vi "Drive Controller.vi"(8 "error in":errorcluster) -> ()   [LabVIEW 2019]
doc: "This VI executes continuously carrying out the current operation and responding to updates or new operation requests. It will often contain the timing or control code that is difficult to place directly in TeleOp. This VI generally opens all sensors and motors and isolates the rest of the robot code from knowing implementation details of how the operations are carried out."
uses:
  <vilib>/Rock Robotics/WPI/Framework/Completion Status.ctl
  Drive Setpoints.ctl
  Drive Operations.ctl
  Dawgma Programming Library/Controls/PurePursuit/RobotNeededPathData.ctl
  <vilib>/Rock Robotics/WPI/ThirdParty/REV Robotics/SPARK MAX/Typedef/Spark MAX Sensor Type.ctl
  <vilib>/Rock Robotics/WPI/ThirdParty/REV Robotics/SPARK MAX/Typedef/Spark MAX Idle Mode.ctl
  <vilib>/Rock Robotics/WPI/DriverStation/WPI_DriverStationRobotMode2.ctl
  <vilib>/Rock Robotics/WPI/ThirdParty/REV Robotics/SPARK MAX/Typedef/Spark MAX Control Type.ctl
  Dawgma Programming Library/Controls/PurePursuit/PathFileData.ctl
  Framework/Robot Global Data.vi
  <vilib>/Rock Robotics/Network Tables/NT Write Numeric Array.vi
  <vilib>/Rock Robotics/Network Tables/NT Read Number.vi
  Configuration/Constants.vi
  <vilib>/Rock Robotics/WPI/ThirdParty/Sensors/navX/_Processing Loop/FRIC_navX_Internal_SPI_ProcessingLoop.vi
  <extravilib>/ChannelInstances/Lossy Stream-c(dbl,dbl,dbl,dbl,dbl,c(dbl,dbl)).lvlib
panel:
  in  "R L & A":bool
  out "Graph":cluster{cluster{"x":dbl, "y":dbl}[]}[](graph)
  in  "PurePursuit Gains":T1={"FFV"=0.0055, "FFA"=0.0025, "Vel PID"={"P"=0.0001, "I"=0.0, "D"=0.0}}
  in  "SensorData":T2={"LeftDistance"=3962.033502451172, "RightDistance"=3821.920006201172, "LeftVelocity"=0.0, "RightVelocity"=0.0, "Angle"=-59.4, "Location"={597.0445781606653, 278.6835922961287}}
  in  "Reset PID":bool
  out "Right Motor Out":dbl=0.05499435407574694
  out "Left Motor Out":dbl=0.05499435407574694
  in  "SparkMAX PID":T3={"P"=0.038, "I"=0.0, "D"=0.0, "F"=0.001, "I Zone"=0.0, "Min Output"=-0.8, "Max Output"=0.8}
  in  "Reset Encoders":bool
  in  "Coast?":bool
  in  "Interactive Values":T4={"Operation"=enum."Drive for Distance", "Left Setpoint"=0.2, "Right Setpoint"=-0.2, "Duration"=0.1, "Distance"=200.0, "RobotNeededPathData"={"Path"=[], "MaxVel"=0.0, "MaxAccel"=0.0, "Backwards?"=FALSE, "PointSpacing"=0.0, "LookaheadDist"=0.0, "Speed/Curve"=1.8, "SlowDistanceAtEnd"=12.0, "SlowSpeed"=15.0, "MaxDeAccel"=0.0}, "PathPath"=""} {"RobotNeededPathData"."SlowSpeed" format="%#_13g"; "RobotNeededPathData"."SlowDistanceAtEnd" format="%#_13g"; "RobotNeededPathData"."Speed/Curve" format="%#_13g"}
  in  "Buttons":cluster{"Execute Cmd":bool, "Abort Cmd":bool}
  out "Command Timing":cluster{"Start Time (ms)":u32, "Iterations":i32}={"Start Time (ms)"=608665, "Iterations"=0}
  out "Status":T7
  out "Current\nCmd":string="Started at  13:49:29.041\nDefault: Reserve,  L 0.0, R 0.0, D 0.000000"
  # "Interactive Command: You may fill in the settings for a command\nand schedule it with the Execute button. You can observe and abort\nany command while fine tuning the code for the controller."
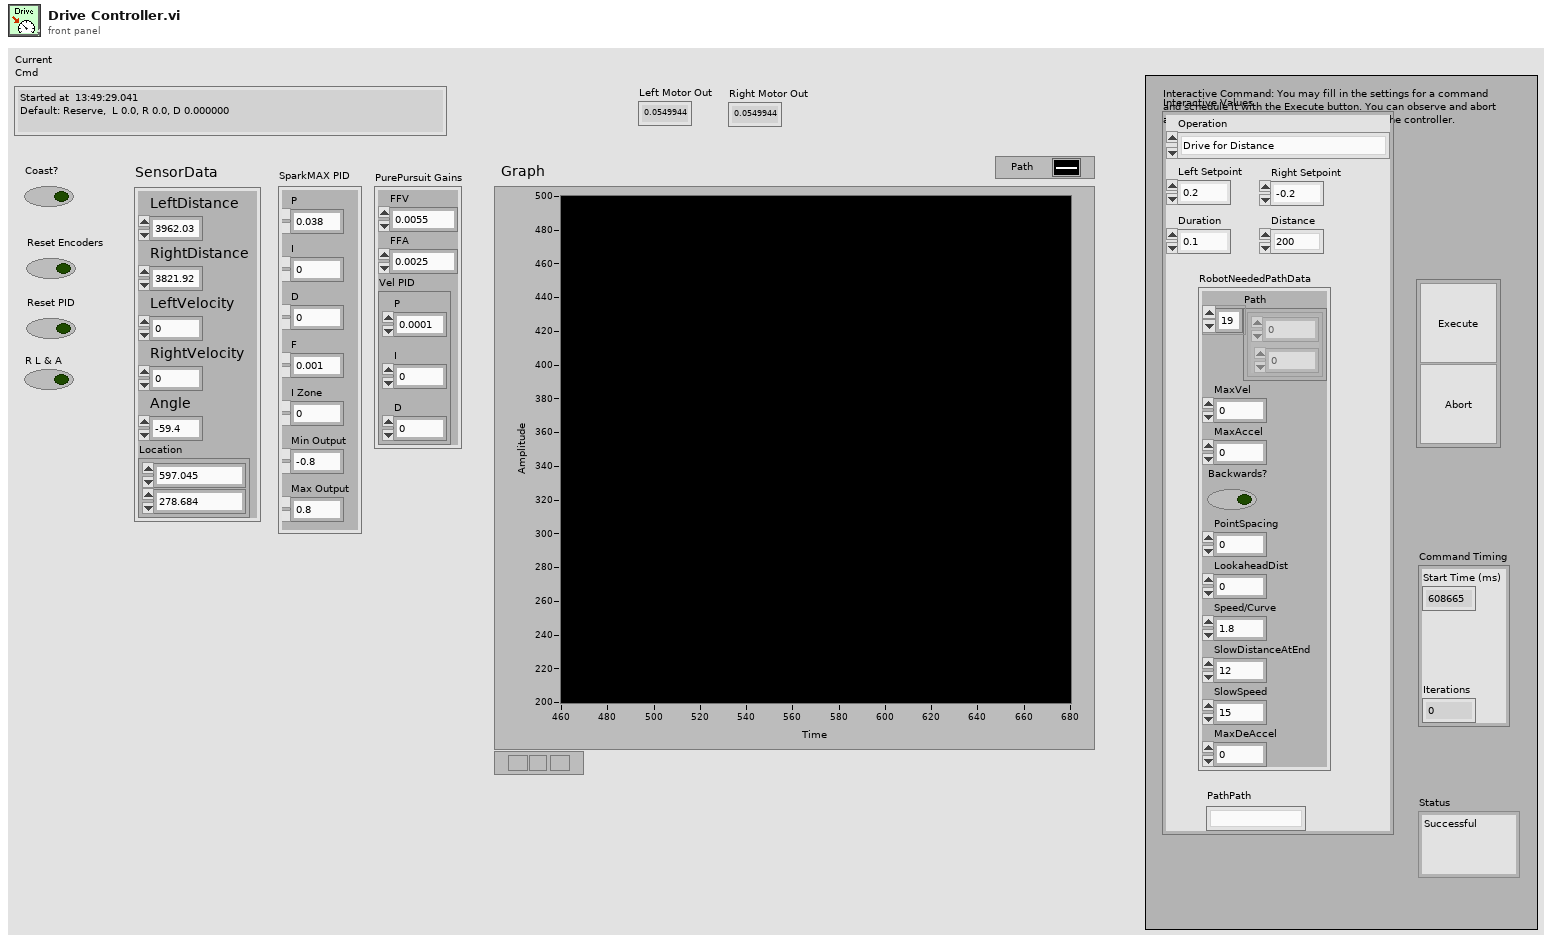
[diagram p1: front panel]
types:
  T1 = cluster{"FFV":dbl, "FFA":dbl, "Vel PID":cluster{"P":dbl, "I":dbl, "D":dbl}}
  T2 = cluster{"LeftDistance":dbl, "RightDistance":dbl, "LeftVelocity":dbl, "RightVelocity":dbl, "Angle":dbl, "Location":cluster{dbl, dbl}}
  T3 = cluster{"P":dbl, "I":dbl, "D":dbl, "F":dbl, "I Zone":dbl, "Min Output":dbl, "Max Output":dbl}
  T4 = typedef "Drive Setpoints.ctl" = cluster{"Operation":T5, "Left Setpoint":dbl, "Right Setpoint":dbl, "Duration":dbl, "Distance":dbl, "RobotNeededPathData":T6, "PathPath":string}
  T5 = typedef "Drive Operations.ctl" = enum16{"Reserve", "Read Current", "Immediate", "Drive for Time", "Drive for Distance", "Drive Path", "Pure Pursuit Test", "Auto Align"}
  T6 = typedef "RobotNeededPathData.ctl" = cluster{"Path":cluster{dbl, dbl}[], "MaxVel":dbl, "MaxAccel":dbl, "Backwards?":bool, "PointSpacing":dbl, "LookaheadDist":dbl, "Speed/Curve":dbl, "SlowDistanceAtEnd":dbl, "SlowSpeed":dbl, "MaxDeAccel":dbl}
  T7 = typedef "Completion Status.ctl" = enum16{"Successful", "Aborted", "Incomplete"}
  T8 = typedef "Spark MAX Idle Mode.ctl" = enum16{"Coast", "Brake"}
  T9 = typedef "Spark MAX Sensor Type.ctl" = enum16{"No Sensor", "Hall Sensor", "Encoder", "-Not Available-", "Analog", "Alternate Encoder"}
  T10 = typedef "WPI_MotorControlDeviceRef.ctl" = cluster{"DeviceStatus":errorcluster, "Type":T11, "PWM":cluster{"PWM Channel":T12, "DeadBand":T13}, "CAN":cluster{"Device Number":u8, "SetOutput VI Ref":variant, "GetOutput VI Ref":variant, "Enable VI Ref":variant, "Disable VI Ref":variant, "Data":variant}, "Invert":bool, "DIO PWM":cluster{"PWM \"Enable\" Channel":T12, "DIOChannel":T14, "PWM Rate":dbl}}
  T11 = typedef "WPI_MotorControlType.ctl" = enum16{"PWM", "CAN", "DIO PWM"}
  T12 = typedef "FPGA_DIOPWMChannel.ctl" = enum8{"PWM 0", "PWM 1", "PWM 2", "PWM 3", "PWM 4", "PWM 5", "PWM 6", "PWM 7", "PWM 8", "PWM 9", "PWM MXP 0", "PWM MXP 1", "PWM MXP 2", "PWM MXP 3", "PWM MXP 4", "PWM MXP 5", "PWM MXP 6", "PWM MXP 7", "PWM MXP 8", "PWM MXP 9", "Invalid"}
  T13 = typedef "WPI_PWMDeadband.ctl" = cluster{"Name":string, "maxPositivePwm":i32, "minPositivePwm":i32, "centerPwm":i32, "maxNegativePwm":i32, "minNegativePwm":i32, "angularRange":u16}
  T14 = typedef "FPGA_DIOChannel.ctl" = enum8{"DIO 0", "DIO 1", "DIO 2", "DIO 3", "DIO 4", "DIO 5", "DIO 6", "DIO 7", "DIO 8", "DIO 9", "DIO MXP 0", "DIO MXP 1", "DIO MXP 2", "DIO MXP 3", "DIO MXP 4", "DIO MXP 5", "DIO MXP 6", "DIO MXP 7", "DIO MXP 8", "DIO MXP 9", "DIO MXP 10", "DIO MXP 11", "DIO MXP 12", "DIO MXP 13", "DIO MXP 14", "DIO MXP 15", "SPI Port CS1", "SPI Port CS2", "SPI Port CS3", "SPI Port MISO", "SPI Port MOSI", "Invalid"}
  T15 = typedef "Command Status Info.ctl" = cluster{"Name":string, "Status":T7, "notifier out":T16}
  T16 = typedef "Completion Notifier.ctl" = refnum<notifier>
  T17 = cluster{"SubSystem Data":T4, cluster{"Start Time (ms)":u32, "Iterations":i32}, cluster{"Command Info":T15, "Description":string, "Default Command":T4, "queue out":refnum<queue>, "Subsystem Name":string}}
  T18 = typedef "WPI_DriverStationRobotMode2.ctl" = enum16{"Autonomous Disabled", "Autonomous Enabled", "Teleop Disabled", "Teleop Enabled", "Disconnected", "Finish", "Test Disabled", "Test Enabled", "Emergency Stopped"}
  T19 = cluster{"Yaw":dbl, "Roll":dbl, "Pitch":dbl, "Heading":dbl, "Fused Heading":dbl}
  T20 = typedef "Spark MAX Control Type.ctl" = enum16{"Percent VBus", "Voltage", "Velocity", "Position", "Smart Motion", "Current", "Smart Velocity"}
  T21 = typedef "PathFileData.ctl" = cluster{"RobotNeeded":T6, "Meta":cluster{"Path (px)":cluster{i32, i32}[], "RobotWidth":dbl, "RobotLength":dbl, "CenterOfRotYOffset":dbl, "Roundedness":dbl, "StartingPositionPreset":u32}}
  T22 = cluster{"SubSystem Data":T4, cluster{"Start Time (ms)":u32, "Iterations":i32}, "Default Command Arguments":cluster{"Command Info":T15, "Description":string, "Default Command":T4, "queue out":refnum<queue>, "Subsystem Name":string}}
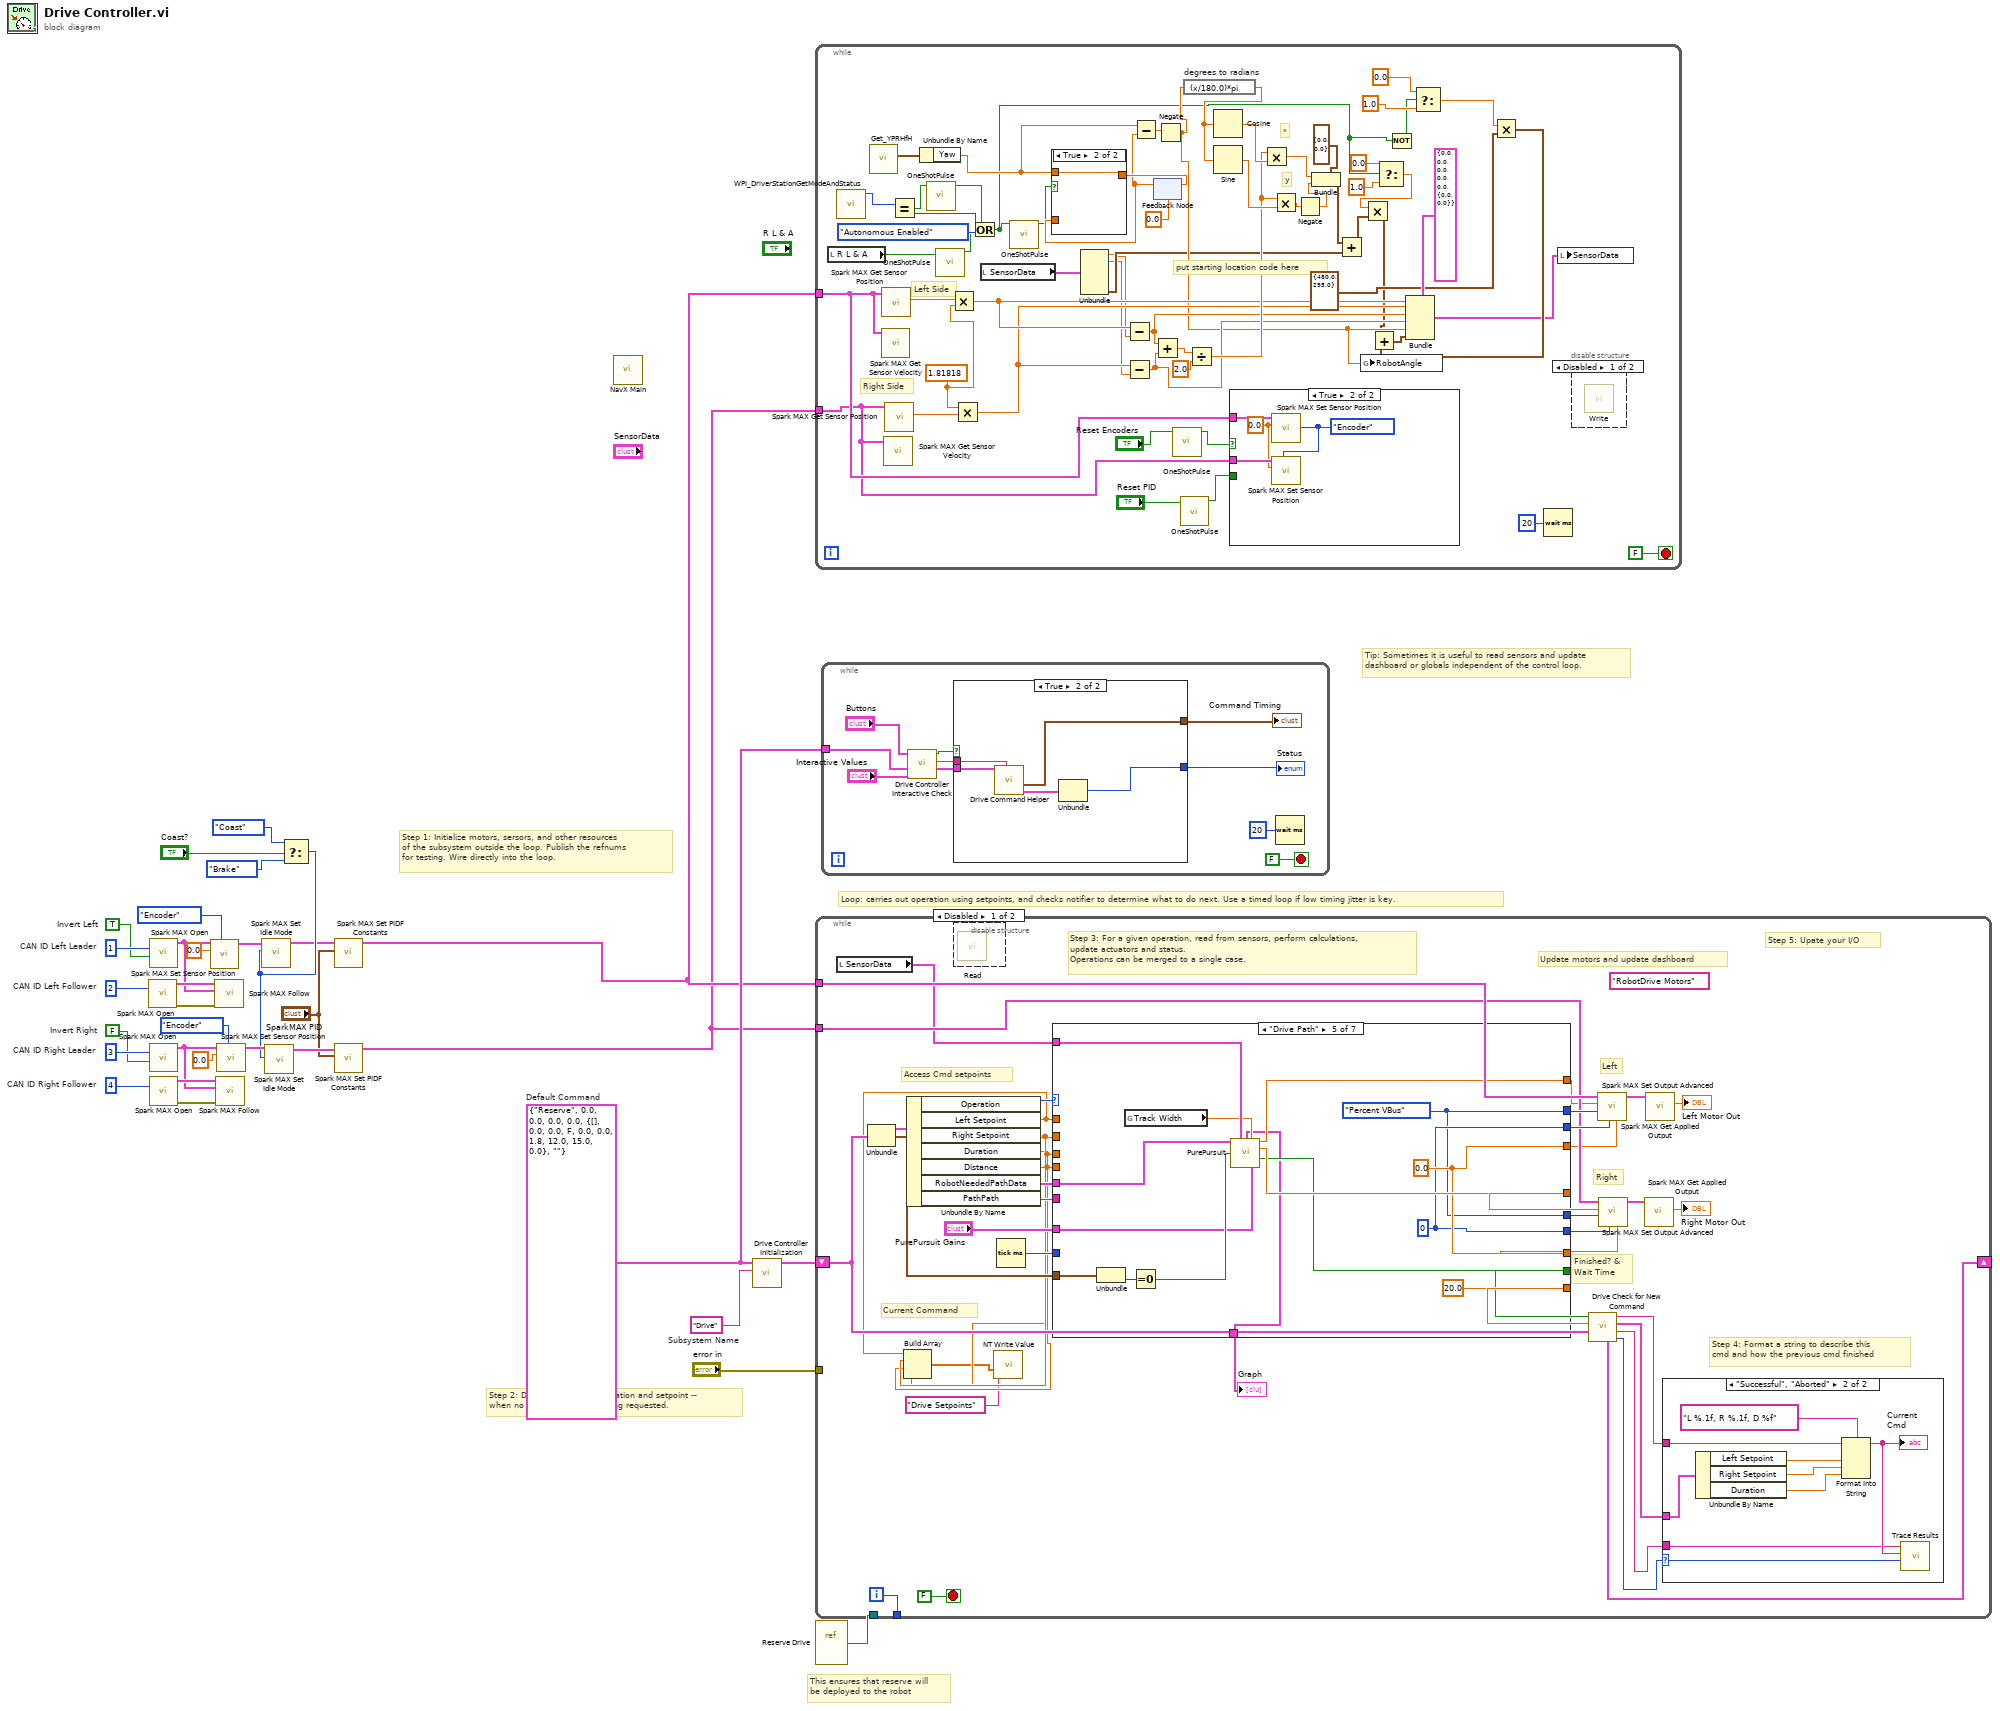
[diagram p0: block diagram]
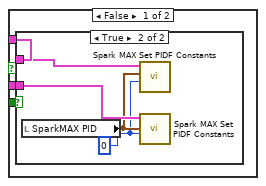
[diagram p4: hidden frame]
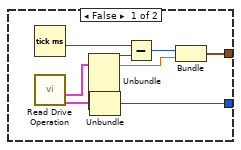
[diagram p6: hidden frame]
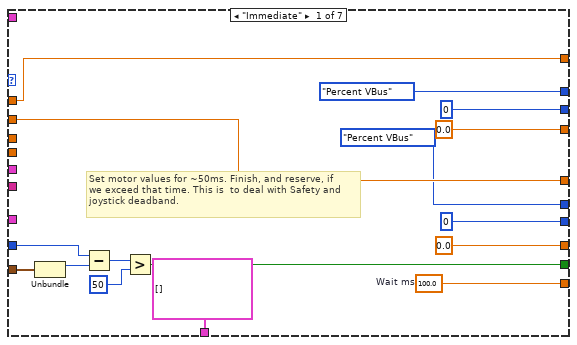
[diagram p9: hidden frame]
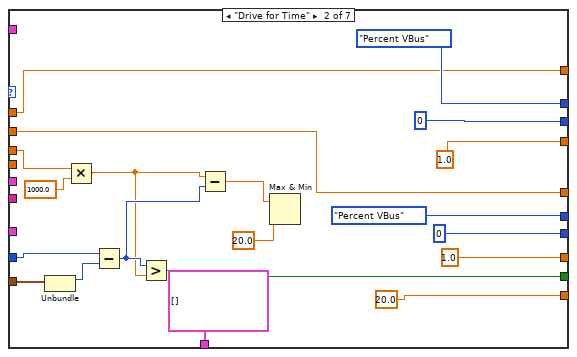
[diagram p10: hidden frame]
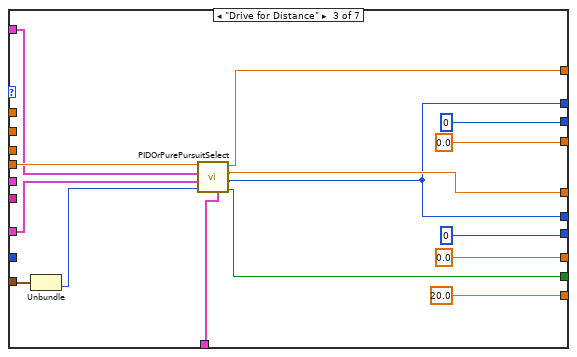
[diagram p11: hidden frame]
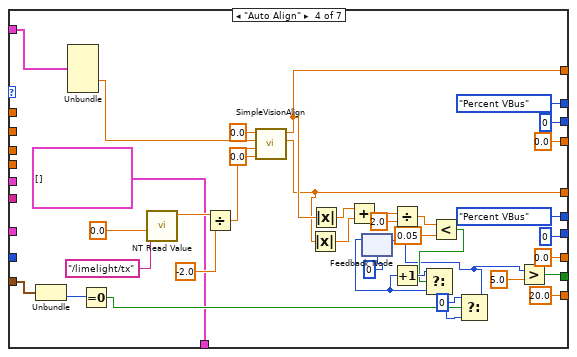
[diagram p12: hidden frame]
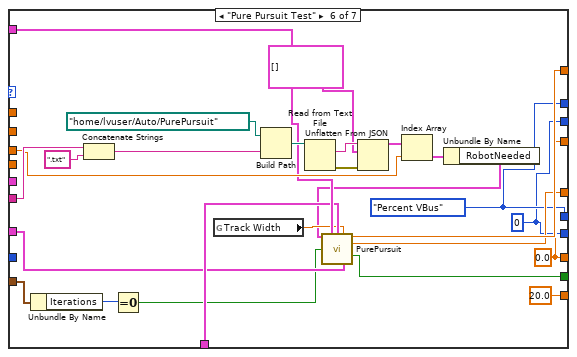
[diagram p13: hidden frame]
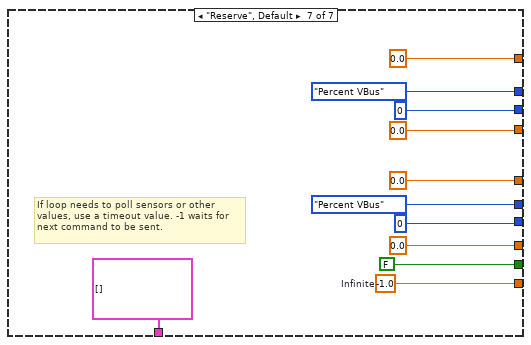
[diagram p14: hidden frame]
diagram:
  w18 = TRUE  # Invert Left
  w19 = FALSE  # Invert Right
  w21 = u8 3  # CAN ID Right Leader
  w20 = u8 4  # CAN ID Right Follower
  w26 = u8 1  # CAN ID Left Leader
  w27 = u8 2  # CAN ID Left Follower
  w28 = T4 {"Operation"=enum."Reserve", "Left Setpoint"=0.0, "Right Setpoint"=0.0, "Duration"=0.0, "Distance"=0.0, "RobotNeededPathData"={"Path"=[], "MaxVel"=0.0, "MaxAccel"=0.0, "Backwards?"=FALSE, "PointSpacing"=0.0, "LookaheadDist"=0.0, "Speed/Curve"=1.8, "SlowDistanceAtEnd"=12.0, "SlowSpeed"=15.0, "MaxDeAccel"=0.0}, "PathPath"=""}  # Default Command
  w32 = "Drive"  # Subsystem Name
  # "This ensures that reserve will\nbe deployed to the robot"
  # "Tip: Sometimes it is useful to read sensors and update\ndashboard or globals independent of the control loop."
  # "Step 2: Define the default operation and setpoint --\nwhen no other operation is being requested."
  # "Step 1: Initialize motors, sersors, and other resources\nof the subsystem outside the loop. Publish the refnums\nfor testing. Wire directly into the loop."
  # "Loop: carries out operation using setpoints, and checks notifier to determine what to do next. Use a timed loop if low timing jitter is key."
  n1 = call <vilib>:"Spark MAX Open.vi"("Device Number"=w27) -> ("error out"=w24:errorcluster, "MotorControlDeviceRef"=w25:T10)  [unwired: 9 in]
  n2 = call <vilib>:"Spark MAX Open.vi"("Invert"=w18, "Device Number"=w26) -> ("MotorControlDeviceRef"=w17:T10)  [unwired: 8 in, 1 out]
  n3 = call <vilib>:"Spark MAX Open.vi"("Invert"=w19, "Device Number"=w21) -> ("MotorControlDeviceRef"=w12:T10)  [unwired: 8 in, 1 out]
  n4 = call <vilib>:"Spark MAX Open.vi"("Device Number"=w20) -> ("error out"=w23:errorcluster, "MotorControlDeviceRef"=w22:T10)  [unwired: 9 in]
  n5 = call <vilib>:"Spark MAX Set Sensor Position.vi"("Sensor Type (Hall Sensor)"=Spark_MAX_Sensor_Type."Encoder", "Position"=0.0, "MotorControlDeviceRef"=w17) -> ("MotorControlDeviceRef"=w8:T10)  [unwired: 7 in, 1 out]
  n6 = call <vilib>:"Spark MAX Follow.vi"("error in (no error)"=w24, "Master Controller"=w17, "MotorControlDeviceRef"=w25) -> ()  [unwired: 7 in, 2 out]
  n7 = call <vilib>:"Spark MAX Follow.vi"("error in (no error)"=w23, "Master Controller"=w12, "MotorControlDeviceRef"=w22) -> ()  [unwired: 7 in, 2 out]
  n8 = call <vilib>:"Spark MAX Set Sensor Position.vi"("Sensor Type (Hall Sensor)"=Spark_MAX_Sensor_Type."Encoder", "Position"=0.0, "MotorControlDeviceRef"=w12) -> ("MotorControlDeviceRef"=w7:T10)  [unwired: 7 in, 1 out]
  n9 = Select(t=Spark_MAX_Idle_Mode."Coast" ("Idle Mode"), s="Coast?", f=Spark_MAX_Idle_Mode."Brake") -> (s? t:f=w6:T8)
  n10 = call <vilib>:"Spark MAX Set Idle Mode.vi"("Idle Mode"=w6, "MotorControlDeviceRef in"=w8) -> ("MotorControlDeviceRef out"=w5:T10)  [unwired: 8 in, 1 out]
  n11 = call <vilib>:"Spark MAX Set Idle Mode.vi"("Idle Mode"=w6, "MotorControlDeviceRef in"=w7) -> ("MotorControlDeviceRef out"=w3:T10)  [unwired: 8 in, 1 out]
  n12 = call <vilib>:"Spark MAX Set PIDF Constants.vi"("PID Constants"="SparkMAX PID", "MotorControlDeviceRef"=w5) -> ("MotorControlDeviceRef"=w4:T10)  [unwired: 8 in, 1 out]
  n13 = call <vilib>:"Spark MAX Set PIDF Constants.vi"("PID Constants"="SparkMAX PID", "MotorControlDeviceRef"=w3) -> ("MotorControlDeviceRef"=w1:T10)  [unwired: 8 in, 1 out]
  n14 = call-poly <vilib>:"NavX Main.vi"() -> ()  [unwired: 12 in]
  n15 = call "Drive Controller Initialization.vi"("Subsystem Name"=w32, "Default Command"=w28) -> ("Current Command"=w30:T17)  [unwired: 9 in]
  n16 = while {
    tunnel: w4 -> [w85]
    tunnel: w1 -> [w84]
    stop <- FALSE stop-if-true
    w62 = 1.81818 ("y")
    # "put starting location code here"
    # "y"
    # "x"
    # "Right Side"
    # "Left Side"
    n17 = local read "R L & A"() -> (w42:bool)
    n18 = call <vilib>:"WPI_DriverStationGetModeAndStatus.vi"() -> ("Robot Mode"=w81:T18)  [unwired: 10 in, 1 out]
    n19 = call <vilib>:"Get_YPRHfH.vi"() -> ("YRPHfH"=w82:T19)  [unwired: 11 in]
    n20 = call <vilib>:"Spark MAX Get Sensor Velocity.vi"("MotorControlDevRef in"=w85) -> ()  [unwired: 7 in, 4 out]
    n21 = call <vilib>:"Spark MAX Get Sensor Position.vi"("MotorControlDevRef in"=w85) -> ("Sensor Position"=w63:dbl)  [unwired: 7 in, 3 out]
    n22 = call <vilib>:"Spark MAX Get Sensor Velocity.vi"("MotorControlDevRef in"=w84) -> ()  [unwired: 7 in, 4 out]
    n23 = call <vilib>:"Spark MAX Get Sensor Position.vi"("MotorControlDevRef in"=w84) -> ("Sensor Position"=w64:dbl)  [unwired: 7 in, 3 out]
    n24 = Equal?(x=w81, y=WPI_DriverStationRobotMode2."Autonomous Enabled" ("Robot Mode")) -> (x = y?=w41:bool)
    n25 = Unbundle By Name(w82) -> ("Yaw"=w77:dbl)
    n26 = call "OneShotPulse.vi"("Input"=w41) -> ("Output"=w40:bool)  [unwired: 10 in]
    n27 = call "OneShotPulse.vi"("Input"=w42) -> ("Output"=w70:bool)  [unwired: 10 in]
    n28 = Multiply(x=w63, y=w62) -> (x*y=w56:dbl)
    n29 = Multiply(x=w62, y=w64) -> (x*y=w55:dbl)
    n30 = Or(x=w40, y=w70) -> (x .or. y?=w49:bool)
    n31 = local read "SensorData"() -> (w36:T2)
    n32 = call "OneShotPulse.vi"("Input"=w49) -> ("Output"=w71:bool)  [unwired: 10 in]
    n33 = Unbundle(w36) -> ("LeftDistance"=w34:dbl, "RightDistance"=w33:dbl, "Location"=w35:cluster{dbl, dbl})  [unwired: 3 out]
    n34 = Subtract(x=w56, y=w34) -> (x-y=w58:dbl)
    n35 = Subtract(x=w55, y=w33) -> (x-y=w57:dbl)
    n36 = feedback #1(0.0) -> (w76:dbl)
    n37 = case shown="True" w71 {
      tunnel: [w92 w93] -> w78
      tunnel: w77 -> [_ w93]
      tunnel: w76 -> [w92 _]
      frame False {
      }
      frame True {
      }
    }
    n38 = Subtract(x=w77, y=w76) -> (x-y=w53:dbl)
    n39 = feedback-in #1(w78) -> ()
    n40 = Add(x=w58, y=w57) -> (x+y=w61:dbl)
    n41 = Negate(x=w53) -> (-x=w52:dbl)
    n42 = call "OneShotPulse.vi"("Input"="Reset Encoders") -> ("Output"=w86:bool)  [unwired: 10 in]
    n43 = call "OneShotPulse.vi"("Input"="Reset PID") -> ("Output"=w88:bool)  [unwired: 10 in]
    n44 = expression code="(x/180.0)*pi" "degrees to radians"(w52) -> (w65:dbl)
    n45 = Divide(x=w61, y=2.0) -> (x/y=w59:dbl)
    n46 = Cosine(x=w65) -> (cos(x)=w74:dbl)
    n47 = Sine(x=w65) -> (sin(x)=w75:dbl)
    n48 = case shown="True" w86 {
      tunnel: w85 -> [w96 w104]
      tunnel: w84 -> [w95 w103]
      tunnel: w88 -> [w94 _]
      frame False {
        n49 = case shown="True" w94 {
          tunnel: w96 -> [_ w100]
          tunnel: w95 -> [_ w99]
          frame False {
          }
          frame True {
            w97 = 0
            n50 = local read "SparkMAX PID"() -> (w98:T3)
            n51 = call <vilib>:"Spark MAX Set PIDF Constants.vi"("PIDF Slot"=w97, "PID Constants"=w98, "MotorControlDeviceRef"=w100) -> ()  [unwired: 7 in, 2 out]
            n52 = call <vilib>:"Spark MAX Set PIDF Constants.vi"("PIDF Slot"=w97, "PID Constants"=w98, "MotorControlDeviceRef"=w99) -> ()  [unwired: 7 in, 2 out]
          }
        }
      }
      frame True {
        w102 = Spark_MAX_Sensor_Type."Encoder" ("Sensor Type (Hall Sensor)")
        w101 = 0.0 ("Position")
        n53 = call <vilib>:"Spark MAX Set Sensor Position.vi"("Sensor Type (Hall Sensor)"=w102, "Position"=w101, "MotorControlDeviceRef"=w104) -> ()  [unwired: 7 in, 2 out]
        n54 = call <vilib>:"Spark MAX Set Sensor Position.vi"("Sensor Type (Hall Sensor)"=w102, "Position"=w101, "MotorControlDeviceRef"=w103) -> ()  [unwired: 7 in, 2 out]
      }
    }
    n55 = Multiply(x=w59, y=w74) -> (x*y=w54:dbl)
    n56 = Multiply(x=w59, y=w75) -> (x*y=w39:dbl)
    n57 = Negate(x=w39) -> (-x=w38:dbl)
    n58 = Bundle(cluster=cluster{dbl, dbl} {0.0, 0.0} ("Location"), w54, w38) -> (w72:cluster{dbl, dbl})
    n59 = Add(x=w72, y=w35) -> (x+y=w69:cluster{dbl, dbl})
    n60 = global write "Robot Global Data.vi" "RobotAngle"(w52) -> ()
    n61 = Select(t=0.0, s=w49, f=1.0) -> (s? t:f=w66:dbl)
    n62 = Multiply(x=w66, y=w69) -> (x*y=w44:cluster{dbl, dbl})
    n63 = Not(x=w49) -> (.not. x?=w48:bool)
    n64 = Select(t=0.0 ("f"), s=w48, f=1.0 ("t")) -> (s? t:f=w47:dbl)
    n65 = Multiply(x=w47, y=cluster{dbl, dbl} {480.0, 295.0}) -> (x*y=w45:cluster{dbl, dbl})
    n66 = Add(x=w44, y=w45) -> (x+y=w43:cluster{dbl, dbl})
    n67 = Bundle(cluster=T2 {"LeftDistance"=0.0, "RightDistance"=0.0, "LeftVelocity"=0.0, "RightVelocity"=0.0, "Angle"=0.0, "Location"={0.0, 0.0}} ("SensorData"), "LeftDistance"=w56, "RightDistance"=w55, "LeftVelocity"=w58, "RightVelocity"=w57, "Angle"=w52, "Location"=w43) -> (w37:T2)
    n68 = Wait (ms)(milliseconds to wait=u32 20) -> ()  [unwired: 1 out]
    n69 = local write "SensorData"(w37) -> ()
    n70 = disable-structure shown="Disabled" {
      frame Disabled {
        n71 = call <extravilib>:"Write.vi"() -> ()  [unwired: 9 in, 3 out]
      }
      frame Enabled {
      }
    }
  }
  n72 = vi-ref "Reserve Drive.vi"() -> (w29:refnum<vi>)
  n73 = while {
    shift-right: [w137] -> _
    shift-left: w30 -> [w130]
    tunnel: [w142] -> _
    tunnel: "error in" -> [_]
    tunnel: w29 -> [_]
    tunnel: w1 -> [w123]
    tunnel: w4 -> [w124]
    i -> [w142]
    stop <- FALSE stop-if-true
    (unwired) "RobotDrive Motors" ("Name")
    # "Right"
    # "Left"
    # "Step 5: Upate your I/O"
    # "Step 4: Format a string to describe this\ncmd and how the previous cmd finished"
    # "Current Command"
    # "Update motors and update dashboard"
    # "Access Cmd setpoints"
    # "Finished? &\nWait Time"
    # "Step 3: For a given operation, read from sensors, perform calculations,\nupdate actuators and status.\nOperations can be merged to a single case."
    n74 = local read "SensorData"() -> (w105:T2)
    n75 = Unbundle(w130) -> ("SubSystem Data"=w141:T4, w131:cluster{"Start Time (ms)":u32, "Iterations":i32})  [unwired: 1 out]
    n76 = Unbundle By Name(w141) -> ("Operation"=w140:T5, "Left Setpoint"=w111:dbl, "Right Setpoint"=w110:dbl, "Duration"=w109:dbl, "Distance"=w108:dbl, "RobotNeededPathData"=w114:T6, "PathPath"=w112:string)
    n77 = Build Array(w111, w110, w109, w108) -> (w107:dbl[])
    n78 = disable-structure shown="Disabled" {
      frame Disabled {
        n79 = call <extravilib>:"Read.vi"() -> ()  [unwired: 6 in, 6 out]
      }
      frame Enabled {
      }
    }
    n80 = call-poly <vilib>:"NT Write Value.vi"("Numeric Array"=w107, "Name"="Drive Setpoints") -> ()  [unwired: 9 in, 1 out]
    n81 = Tick Count (ms)() -> (millisecond timer value=w139:u32)
    n82 = case shown="\"Drive Path\"" w140 {
      tunnel: [w168 20.0 ("y") 20.0 ("Infinite") 20.0 ("Infinite") 20.0 ("Infinite") 20.0 ("Infinite") w292] -> w136
      tunnel: [w163 w181 w192 w223 w248 w267 FALSE ("ignore previous (F)")] -> w135
      tunnel: w131 -> [w162 w186 w198 w210 w254 w261 _]
      tunnel: w111 -> [w161 w183 _ _ _ _ _]
      tunnel: w110 -> [w160 w182 _ _ _ _ _]
      tunnel: w109 -> [_ w177 _ _ _ w273 _]
      tunnel: w139 -> [w164 w184 _ _ _ _ _]
      tunnel: [w161 w183 w195 w221 w250 w269 0.0 ("Left Setpoint")] -> w122
      tunnel: [w160 w182 w194 w220 w249 w268 0.0 ("Right Setpoint")] -> w120
      tunnel: [Spark_MAX_Control_Type."Percent VBus" ("Control Mode") Spark_MAX_Control_Type."Percent VBus" ("Control Mode") w193 Spark_MAX_Control_Type."Percent VBus" ("Control Mode") w244 w265 Spark_MAX_Control_Type."Percent VBus" ("Control Mode")] -> w129
      tunnel: [Spark_MAX_Control_Type."Percent VBus" ("Control Mode") Spark_MAX_Control_Type."Percent VBus" ("Control Mode") w193 Spark_MAX_Control_Type."Percent VBus" ("Control Mode") w244 w265 Spark_MAX_Control_Type."Percent VBus" ("Control Mode")] -> w128
      tunnel: w108 -> [_ _ w197 _ _ _ _]
      tunnel: [0 ("PIDF Slot (0)") 0 ("PIDF Slot (0)") 0 ("PIDF Slot (0)") 0 ("PIDF Slot (0)") w245 w263 0 ("PIDF Slot (0)")] -> w127
      tunnel: [0 ("PIDF Slot (0)") 0 ("PIDF Slot (0)") 0 ("PIDF Slot (0)") 0 ("PIDF Slot (0)") w245 w263 0 ("PIDF Slot (0)")] -> w126
      tunnel: [0.0 ("Arbitrary Feed Forward (0)") 1.0 ("Arbitrary Feed Forward (0)") 0.0 ("Arbitrary Feed Forward (0)") 0.0 ("Arbitrary Feed Forward (0)") w246 w264 0.0 ("Arbitrary Feed Forward (0)")] -> w125
      tunnel: [0.0 ("Arbitrary Feed Forward (0)") 1.0 ("Arbitrary Feed Forward (0)") 0.0 ("Arbitrary Feed Forward (0)") 0.0 ("Arbitrary Feed Forward (0)") w246 w264 0.0 ("Arbitrary Feed Forward (0)")] -> w121
      tunnel: w105 -> [_ _ w190 w240 w251 w272 _]
      tunnel: "PurePursuit Gains" -> [_ _ w191 _ w241 w262 _]
      tunnel: w114 -> [_ _ _ _ w255 _ _]
      tunnel: [cluster{cluster{"x":dbl, "y":dbl}[]}[] [] ("Graph") cluster{cluster{"x":dbl, "y":dbl}[]}[] [] ("Graph") w189 cluster{cluster{"x":dbl, "y":dbl}[]}[] [] ("Graph") w242 w271 cluster{cluster{"x":dbl, "y":dbl}[]}[] [] ("Graph")] -> w113
      tunnel: w112 -> [_ _ _ _ _ w274 _]
      frame "Immediate" {
        w168 = 100.0  # Wait ms
        # "Set motor values for ~50ms. Finish, and reserve, if\nwe exceed that time. This is  to deal with Safety and\njoystick deadband."
        n83 = Unbundle(w162) -> ("Start Time (ms)"=w165:u32)  [unwired: 1 out]
        n84 = Subtract(x=w164, y=w165) -> (x-y=w166:u32)
        n85 = Greater?(x=w166, y=u8 50 ("Left Motor")) -> (0:w163:bool)
      }
      frame "Drive for Time" {
        n86 = Unbundle(w186) -> ("Start Time (ms)"=w185:u32)  [unwired: 1 out]
        n87 = Multiply(x=w177, y=1000.0) -> (x*y=w176:dbl)
        n88 = Subtract(x=w184, y=w185) -> (x-y=w179:u32)
        n89 = Greater?(x=w179, y=w176) -> (0:w181:bool)
        n90 = Subtract(x=w176, y=w179) -> (x-y=w178:dbl)
        n91 = Max & Min(x=w178, y=20.0) -> ()  [unwired: 2 out]
      }
      frame "Drive for Distance" {
        n92 = Unbundle(w198) -> ("Iterations"=w196:i32)  [unwired: 1 out]
        n93 = call "PIDOrPurePursuitSelect.vi"("Distance"=w197, "SensorData"=w190, "PurePursuit Gains"=w191, "Iterations"=w196) -> ("Graph"=w189:cluster{cluster{"x":dbl, "y":dbl}[]}[], "Left Output"=w195:dbl, "Right Output"=w194:dbl, "Control Mode"=w193:T20, "Done?"=w192:bool)  [unwired: 2 in]
      }
      frame "Auto Align" {
        n94 = Unbundle(w210) -> ("Iterations"=w209:i32)  [unwired: 1 out]
        n95 = Unbundle(w240) -> ("Angle"=w239:dbl)  [unwired: 5 out]
        n96 = Equal To 0?(x=w209) -> (x = 0?=w208:bool)
        n97 = call-poly <vilib>:"NT Read Value.vi"("Default Value"=0.0, "Name"="/limelight/tx") -> ("Numeric"=w236:dbl)  [unwired: 8 in, 1 out]
        n98 = Divide(x=w236, y=-2.0) -> (x/y=w234:dbl)
        n99 = call "SimpleVisionAlign.vi"("Manual Turn"=0.0, "Target Offset"=w234, "Gyro Angle"=w239, "Throttle"=0.0) -> ("Right Power"=w220:dbl, "Left Power"=w221:dbl)  [unwired: 6 in]
        n100 = Absolute Value(x=w220) -> (abs(x)=w219:dbl)
        n101 = Absolute Value(x=w221) -> (abs(x)=w218:dbl)
        n102 = Add(x=w218, y=w219) -> (x+y=w217:dbl)
        n103 = feedback #2(0) -> (w212:i32)
        n104 = Divide(x=w217, y=2.0) -> (x/y=w215:dbl)
        n105 = Increment(x=w212) -> (x+1=w213:i32)
        n106 = Less?(x=w215, y=0.05) -> (x < y?=w211:bool)
        n107 = Select(t=w213, s=w211, f=w212) -> (s? t:f=w206:i32)
        n108 = Select(t=0, s=w208, f=w206) -> (s? t:f=w205:i32)
        n109 = feedback-in #2(w205) -> ()
        n110 = Greater?(x=w205, y=5.0) -> (0:w223:bool)
      }
      frame "Drive Path" {
        w244 = Spark_MAX_Control_Type."Percent VBus" ("Control Mode")
        w245 = 0
        w246 = 0.0
        n111 = Unbundle(w254) -> ("Iterations"=w253:i32)  [unwired: 1 out]
        n112 = global read "Constants.vi" "Track Width"() -> (w243:dbl)
        n113 = Equal To 0?(x=w253) -> (x = 0?=w252:bool)
        n114 = call "PurePursuit.vi"("RobotNeededPathData"=w255, "SensorData"=w251, "Trackwidth"=w243, "Reset"=w252, "Gains"=w241) -> ("Graph"=w242:cluster{cluster{"x":dbl, "y":dbl}[]}[], "LeftValue"=w250:dbl, "RightValue"=w249:dbl, "Done"=w248:bool)  [unwired: 5 in, 2 out]
      }
      frame "Pure Pursuit Test" {
        w265 = Spark_MAX_Control_Type."Percent VBus" ("Control Mode")
        w263 = 0 ("PIDF Slot (0)")
        w264 = 0.0 ("Arbitrary Feed Forward (0)")
        n115 = Unbundle By Name(w261) -> ("Iterations"=w260:i32)
        n116 = Concatenate Strings(w274, ".txt" ("string")) -> (w280:string)
        n117 = Equal To 0?(x=w260) -> (x = 0?=w259:bool)
        n118 = global read "Constants.vi" "Track Width"() -> (w270:dbl)
        n119 = Build Path(base path=path "/home/lvuser/Auto/PurePursuit", name or relative path=w280) -> (appended path=w278:path)
        n120 = Read from Text File(file (use dialog)=w278) -> (text=w276:string, error out=w277:errorcluster)  [unwired: 3 in, 2 out]
        n121 = Unflatten From JSON(JSON string=w276, type and defaults=T21[] [], error in (no error)=w277) -> (value=w256:T21[])  [unwired: 4 in, 1 out]
        n122 = Index Array(array=w256, index=w273) -> (element=w257:T21)
        n123 = Unbundle By Name(w257) -> ("RobotNeeded"=w258:T6)
        n124 = call "PurePursuit.vi"("RobotNeededPathData"=w258, "SensorData"=w272, "Trackwidth"=w270, "Reset"=w259, "Gains"=w262) -> ("Graph"=w271:cluster{cluster{"x":dbl, "y":dbl}[]}[], "LeftValue"=w269:dbl, "RightValue"=w268:dbl, "Done"=w267:bool)  [unwired: 5 in, 2 out]
      }
      frame "Reserve", Default {
        w292 = -1.0  # Infinite
        # "If loop needs to poll sensors or other\nvalues, use a timeout value. -1 waits for\nnext command to be sent."
      }
    }
    "Graph" <- w113
    n125 = call "Drive Check for New Command.vi"("input cluster"=w130, "Wait time (ms)"=w136, "Finished?"=w135) -> ("Completion"=w138:T7, "Subsystem Name"=w132:string, "Current Command"=w133:T4, "Initial Trace String"=w134:string, "Next Command"=w137:T22)  [unwired: 4 in]
    n126 = call <vilib>:"Spark MAX Set Output Advanced.vi"("Arbitrary Feed Forward (0)"=w121, "PIDF Slot (0)"=w127, "Control Mode"=w128, "Setpoint"=w122, "MotorControlDevRef"=w124) -> ("MotorControlDevRef"=w119:T10)  [unwired: 5 in, 1 out]
    n127 = call <vilib>:"Spark MAX Set Output Advanced.vi"("Arbitrary Feed Forward (0)"=w125, "PIDF Slot (0)"=w126, "Control Mode"=w129, "Setpoint"=w120, "MotorControlDevRef"=w123) -> ("MotorControlDevRef"=w117:T10)  [unwired: 5 in, 1 out]
    n128 = call <vilib>:"Spark MAX Get Applied Output.vi"("MotorControlDevRef in"=w117) -> ("Applied Output"=→"Right Motor Out":dbl)  [unwired: 7 in, 3 out]
    n129 = call <vilib>:"Spark MAX Get Applied Output.vi"("MotorControlDevRef in"=w119) -> ("Applied Output"=→"Left Motor Out":dbl)  [unwired: 7 in, 3 out]
    n130 = case shown="\"Successful\", \"Aborted\"" w138 {
      selector: w138 -> [_ w152]
      tunnel: w134 -> [_ w147]
      tunnel: w133 -> [_ w148]
      tunnel: w132 -> [_ w144]
      frame "Incomplete", Default {
        # "Continuing current command"
      }
      frame "Successful", "Aborted" {
        # "Report and setup for next command"
        n131 = Unbundle By Name(w148) -> ("Left Setpoint"=w150:dbl, "Right Setpoint"=w151:dbl, "Duration"=w145:dbl)
        n132 = Format Into String(format string="L %.1f, R %.1f, D %f", initial string=w147, w150, w151, w145) -> (resulting string=w146:string)  [unwired: 1 in, 1 out]
        "Current\nCmd" <- w146
        n133 = call <vilib>:"Trace Results.vi"("Status of previous command"=w152, "Description"=w146, "Subsystem"=w144) -> ()  [unwired: 9 in]
      }
    }
  }
  n134 = while {
    tunnel: w28 -> [w294]
    stop <- FALSE stop-if-true
    n135 = call "Drive Controller Interactive Check.vi"("Interactive Command In"="Interactive Values", "Default Command"=w294, "Buttons"="Buttons") -> ("Interactive Command Out"=w296:T4, "Trace String"=w297:string, "Schedule"=w298:bool)  [unwired: 6 in]
    n136 = case shown="True" w298 {
      tunnel: [w307 w315] -> w299
      tunnel: [w306 w311] -> w300
      tunnel: w297 -> [_ w313]
      tunnel: w296 -> [_ w312]
      frame False {
        n137 = Tick Count (ms)() -> (millisecond timer value=w310:u32)
        n138 = call "Read Drive Operation.vi"() -> ("Command Info"=w304:T15, "SubSystem Data"=w303:T4)  [unwired: 9 in, 1 out]
        n139 = Unbundle(w303) -> ("Operation"=w308:T5, "Left Setpoint"=w305:dbl)  [unwired: 5 out]
        n140 = Unbundle(w304) -> ("Status"=w307:T7)  [unwired: 2 out]
        n141 = Subtract(x=w310, y=w308) -> (x-y=w309:u32)
        n142 = Bundle(w309, "Left Setpoint"=w305) -> (w306:cluster{u32, "Left Setpoint":dbl})  [unwired: 1 in]
      }
      frame True {
        n143 = call "Drive Command Helper.vi"("Description"=w313, "SubSystem Data"=w312) -> ("Command Info Out"=w314:T15, "Command Timing"=w311:cluster{"Start Time (ms)":u32, "Iterations":i32})  [unwired: 7 in, 1 out]
        n144 = Unbundle(w314) -> ("Status"=w315:T7)  [unwired: 2 out]
      }
    }
    "Status" <- w299
    "Command Timing" <- w300
    n145 = Wait (ms)(milliseconds to wait=u32 20) -> ()  [unwired: 1 out]
  }
